vi "CO MFR loff.vi"(7 "Flow rate":dbl, 8 "O2 Eq Up":dbl, 9 "O2 Measured":dbl, 10 "O2t %":dbl, 11 "Lambda_t":dbl) -> (2 "CO MFR":dbl)   [LabVIEW 2014]
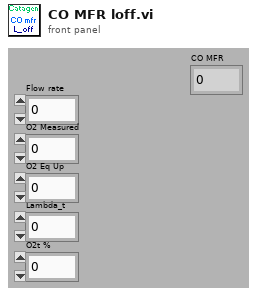
[diagram p1: front panel]
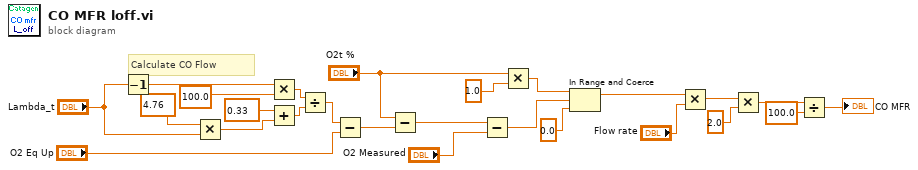
[diagram p0: block diagram]
diagram:
  # "Calculate CO Flow"
  n1 = Decrement(x="Lambda_t") -> (x-1=w25:dbl)
  n2 = Multiply(x=4.76, y="Lambda_t") -> (x*y=w23:dbl)
  n3 = Multiply(x=w25, y=100.0) -> (x*y=w24:dbl)
  n4 = Add(x=0.33, y=w23) -> (x+y=w22:dbl)
  n5 = Divide(x=w24, y=w22) -> (x/y=w12:dbl)
  n6 = Subtract(x=w12, y="O2 Eq Up") -> (x-y=w13:dbl)
  n7 = Subtract(x="O2t %", y=w13) -> (x-y=w15:dbl)
  n8 = Subtract(x=w15, y="O2 Measured") -> (x-y=w10:dbl)
  n9 = Multiply(x="O2t %", y=1.0) -> (x*y=w7:dbl)
  n10 = In Range and Coerce(upper limit=w7, x=w10, lower limit=0.0) -> (coerced(x)=w9:dbl)  [unwired: 1 out]
  n11 = Multiply(x=w9, y="Flow rate") -> (x*y=w14:dbl)
  n12 = Multiply(x=w14, y=2.0) -> (x*y=w20:dbl)
  n13 = Divide(x=w20, y=100.0) -> (x/y=→"CO MFR":dbl)
